vi "prova lv acasa.vi"() -> ()   [LabVIEW 2020]
panel:
  out "x >= y?":bool
  in  "Numeric":dbl
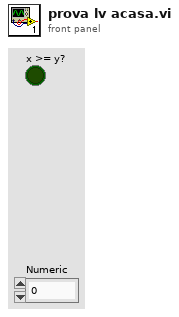
[diagram p1: front panel]
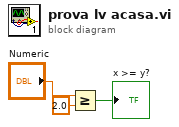
[diagram p0: block diagram]
diagram:
  n1 = Greater Or Equal?(x="Numeric", y=2.0) -> (x >= y?=→"x >= y?":bool)
